vi "IB Panel.vi"() -> ()   [LabVIEW 2015, in "Linearisierung v2.lvlib" / "Gasteiler.lvlib" / "Horiba GDC.lvlib"]
uses:
  Horiba GDC.lvlib
  <vilib>/Instr/_visa.llb/VISA Configure Serial Port (Instr).vi
  Stats.ctl
panel:
  out "Status":T1
  in  "termination char\n(0xA = '\\n' = LF)":u8=13 caption="Endzeichen\n(0xA = '\\n' = LF)" format="%.0x"
  out "error out":errorcluster caption="Fehler (Ausgang)"
  in  "Enable Termination\nChar (T)":bool=TRUE caption="Abschlusszeichen\naktivieren (T)"
  in  "stop bits":u16(ring)=10 caption="Stoppbits (10: 1 Bit)" items=["1.0"=10, "1.5"=15, "2.0"=20]
  in  "data bits":u16=8 caption="Datenbits (8)" min=5 max=8 step=1
  in  "baud rate":u32=9600 caption="Baudrate (9600)"
  in  "timeout":u32=10000 caption="Timeout (10 s)"
  in  "VISA resource name":refnum<visa-resource-name> caption="VISA-Ressourcenname"
  out "Daten":string
  out "Befehl":string
  in  "Daten":string[](array[string])
  in  "Befehl":string
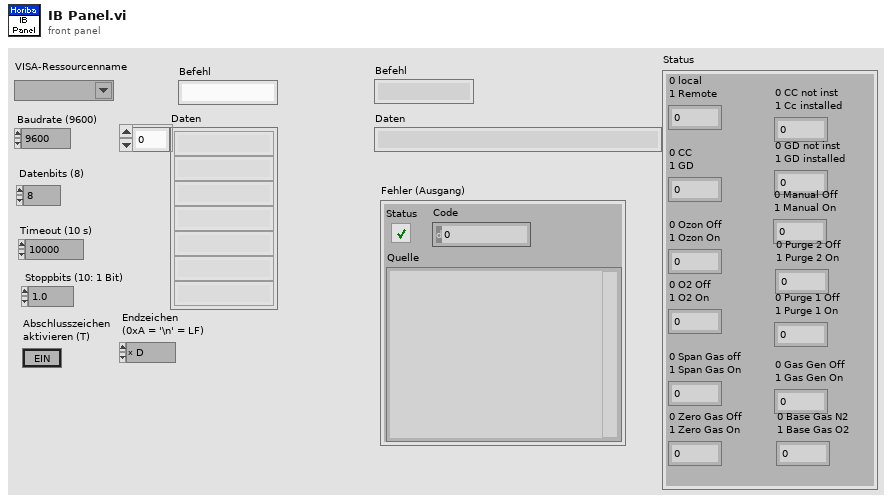
[diagram p1: front panel]
types:
  T1 = typedef "Linearisierung v2.lvlib/Gasteiler.lvlib/Horiba GDC.lvlib/Stats.ctl" = cluster{"0 local\n1 Remote":i16, "0 CC\n1 GD":i16, "0 Ozon Off\n1 Ozon On":i16, "0 O2 Off\n1 O2 On":i16, "0 Span Gas off\n1 Span Gas On ":i16, "0 Zero Gas Off\n1 Zero Gas On":i16, "0 CC not inst\n1 Cc installed":i16, "0 GD not inst\n1 GD installed":i16, "0 Manual Off\n1 Manual On":i16, "0 Purge 2 Off\n1 Purge 2 On":i16, "0 Purge 1 Off\n1 Purge 1 On":i16, "0 Gas Gen Off\n1 Gas Gen On":i16, "0 Base Gas N2\n1 Base Gas O2":i16}
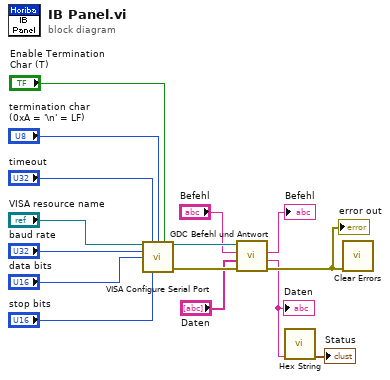
[diagram p0: block diagram]
diagram:
  n1 = call-poly "VISA Configure Serial Port"("VISA resource name"="VISA resource name", "timeout (10sec)"="timeout", "termination char\n(0xA = '\\n' = LF)"="termination char\n(0xA = '\\n' = LF)", "Enable Termination\nChar (T)"="Enable Termination\nChar (T)", "baud rate (9600)"="baud rate", "data bits (8)"="data bits", "stop bits (10: 1 bit)"="stop bits") -> ("VISA resource name out"=w15:refnum<visa-resource-name>, "error out"=w14:errorcluster)  [unwired: 7 in]
  n2 = call "GDC Befehl und Antwort.vi"("error in (no error)"=w14, "Daten"="Daten", "Befehl"="Befehl", "VISA-Ressourcenname"=w15) -> ("error out"=w4:errorcluster, "Daten"=w2:string, "Befehl"=→"Befehl":string)  [unwired: 4 in, 1 out]
  "Daten" <- w2
  "error out" <- w4
  n3 = call "Hex String.vi"("Eingabe String"=w2) -> ("Status"=→"Status":T1)  [unwired: 10 in]
  n4 = call <vilib>:"Clear Errors.vi"("error in (no error)"=w4) -> ()  [unwired: 5 in, 2 out]
